vi "InitFromXML.vi"(8 "error in (no error)":errorcluster, 10 "XML":string, 11 "Help in":refnum<class "Help.lvclass">) -> (0 "error out":errorcluster, 3 "Help out":refnum<class "Help.lvclass">)   [LabVIEW 2009, in "NavScreen.lvlib" / "Help.lvclass"]
uses:
  Help.lvclass
  ClickableText/ClickableText.lvclass
  Help.lvclass/Help.ctl
  NavScreen.lvlib
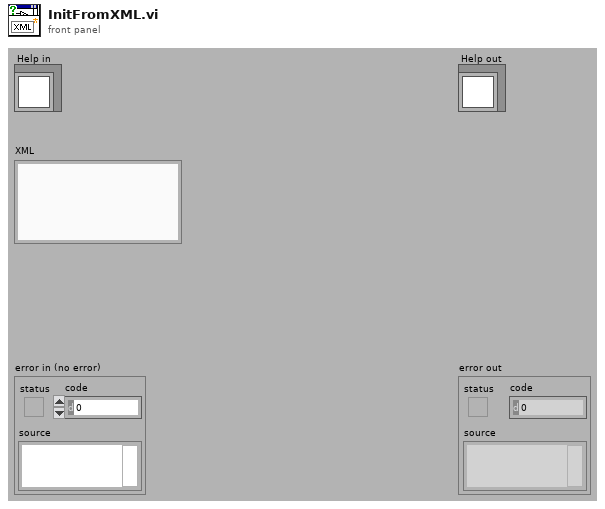
[diagram p1: front panel]
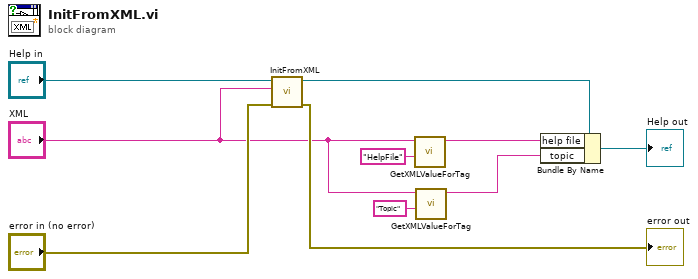
[diagram p0: block diagram]
diagram:
  n1 = call-parent "InitFromXML.vi"("error in (no error)"="error in (no error)", "XML"="XML", "ClickableText in"="Help in") -> ("error out"=→"error out":errorcluster, "ClickableText out"=w10:refnum<class "Help.lvclass">)  [unwired: 7 in]
  n2 = call "GetXMLValueForTag.vi"("tag"="HelpFile", "XML"="XML") -> ("value"=w5:string)  [unwired: 8 in, 1 out]
  n3 = call "GetXMLValueForTag.vi"("tag"="Topic", "XML"="XML") -> ("value"=w1:string)  [unwired: 8 in, 1 out]
  n4 = Bundle By Name(cluster=w10, "help file"=w5, "topic"=w1) -> (→"Help out":refnum<class "Help.lvclass">)
